vi "Create Enumerations.vi"(7 "App":refnum<vi>, 8 "error in (no error)":errorcluster, 11 "LV-Protoc in":refnum<class "LV-Protoc.lvclass">) -> (0 "error out":errorcluster, 3 "LV-Protoc out":refnum<class "LV-Protoc.lvclass">)   [LabVIEW 2020, in "LV-Protoc.lvlib" / "LV-Protoc.lvclass"]
uses:
  LV-Protoc.lvclass
  LV-Protoc.lvclass/LV-Protoc.ctl
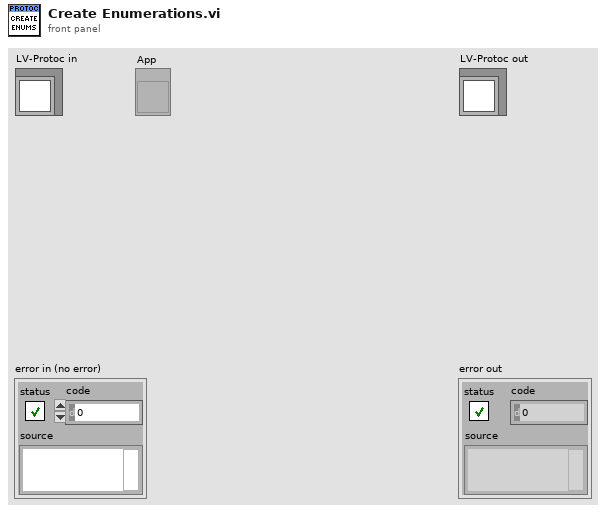
[diagram p1: front panel]
types:
  T1 = typedef "LV-Proto.lvlib/Enumeration.ctl" = cluster{"Name":string, "Values":T2[], "Reserved Numbers":u32[], "Reserved Names":string[]}
  T2 = typedef "LV-Proto.lvlib/Enum Value.ctl" = cluster{"Name":string, "Value":i32}
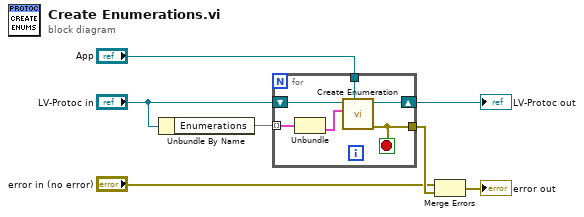
[diagram p0: block diagram]
diagram:
  n1 = Unbundle By Name("LV-Protoc in") -> ("Enumerations"=w7:map{string, T1})
  n2 = for {
    tunnel: w7 -> [w12] mode=indexing
    shift-right: [w10] -> w5
    shift-left: "LV-Protoc in" -> [w13]
    tunnel: [w9] -> w4
    tunnel: "App" -> [w8]
    stop <- w9 stop-if-true
    n3 = Unbundle(w12) -> ("Enumeration"=w11:T1)  [unwired: 1 out]
    n4 = call "Create Enumeration.vi"("App"=w8, "Enumeration"=w11, "LV-Protoc in"=w13) -> ("error out"=w9:errorcluster, "LV-Protoc out"=w10:refnum<class "LV-Protoc.lvclass">)  [unwired: 7 in]
  }
  "LV-Protoc out" <- w5
  n5 = Merge Errors("error in (no error)", w4) -> (→"error out":errorcluster)
